vi "_script_execute.vi"(4 "QD Plugins Dir":path, 6 "QD Text":string, 8 "error in (no error)":errorcluster, 9 "Shift?":bool, 10 "Focus":enum8{"FP", "BD"}(ring), 11 "VI Refnum":refnum<vi>) -> (0 "error out":errorcluster)   [LabVIEW 2019, in "Script.lvlib"]
doc: "Executes scripts shortcuts defined in the Quick Drop arguments.\n\nHelp: Ctrl-Space + \"?\" + Ctrl-S\n\nCreated by: Ryan Pacini"
uses:
  Script.lvlib
  _script_defs.ctl
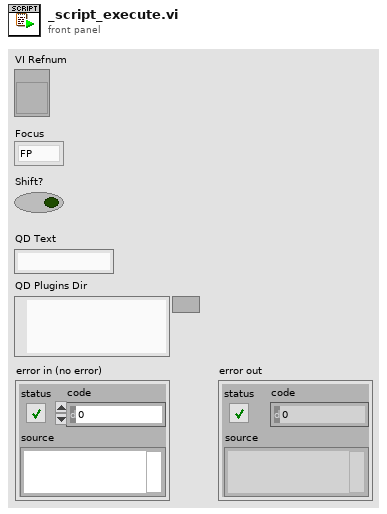
[diagram p1: front panel]
types:
  T1 = typedef "Script.lvlib/_script_defs.ctl" = cluster{"plugins":cluster{"vi":path, "desc":string}[], "defaults":cluster{"uid":string, "name":string}[], "shortcuts":cluster{"shortcut":string, "uids":string[]}[], "defaults?":bool}
  T2 = enum16{"open", "replace", "create", "open or create", "replace or create", "replace or create with confirmation"}
  T3 = cluster{"name":string, "default":cluster{"uid":string, "name":string}}
  T4 = cluster{"name":string, "default":cluster{"uid":string, "name":string}}[]
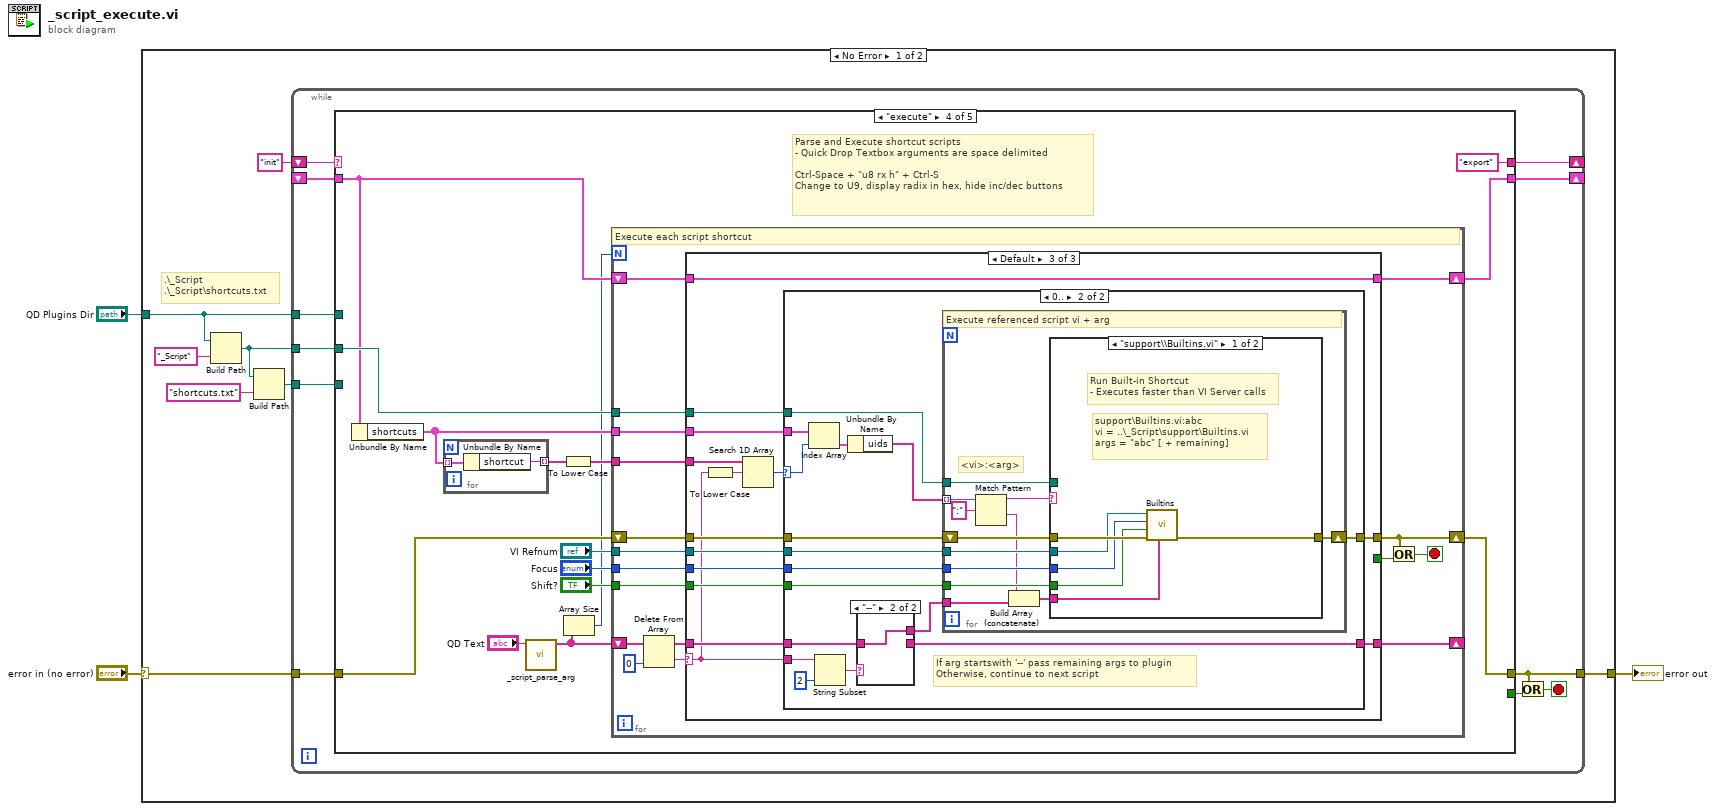
[diagram p0: block diagram]
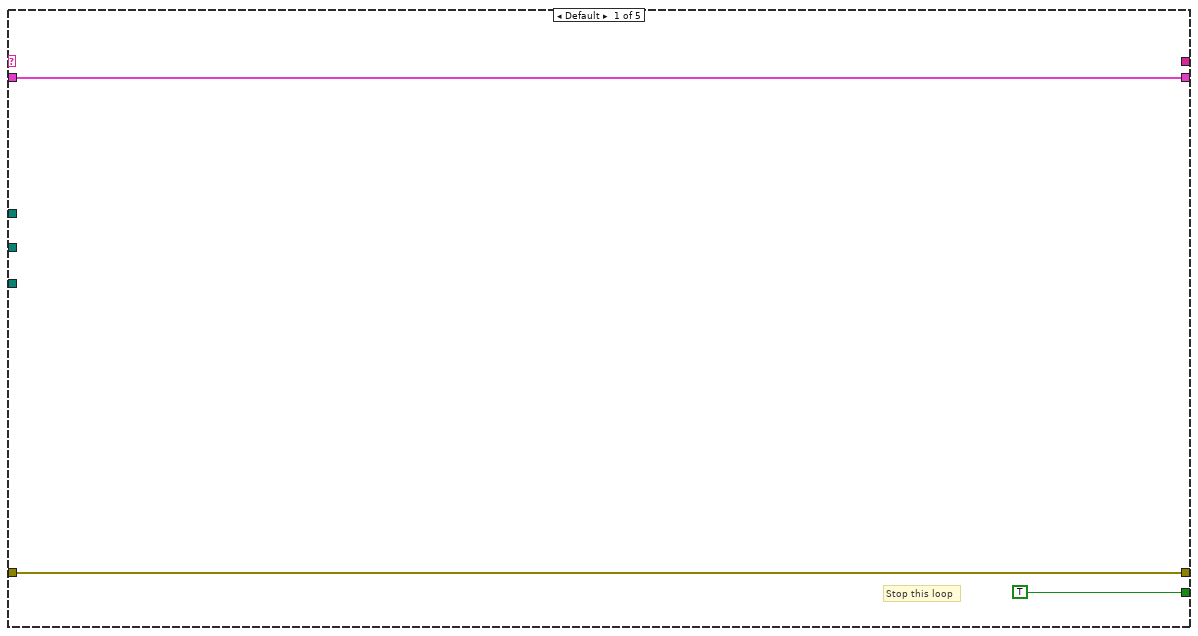
[diagram p2: hidden frame]
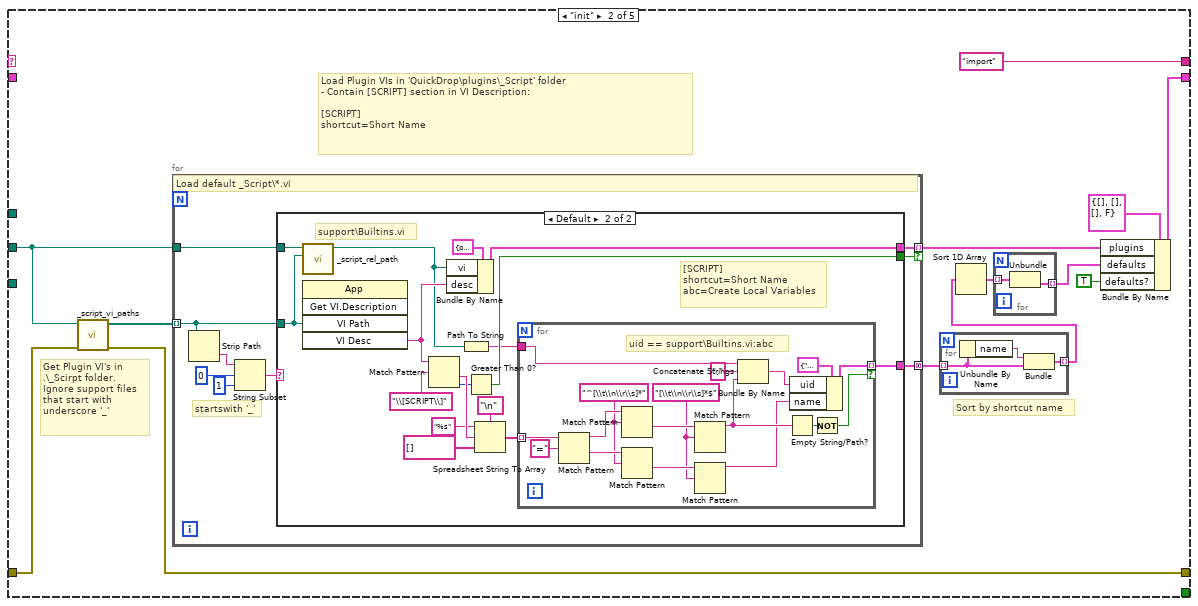
[diagram p3: hidden frame]
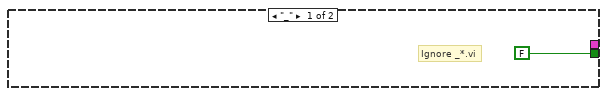
[diagram p4: hidden frame]
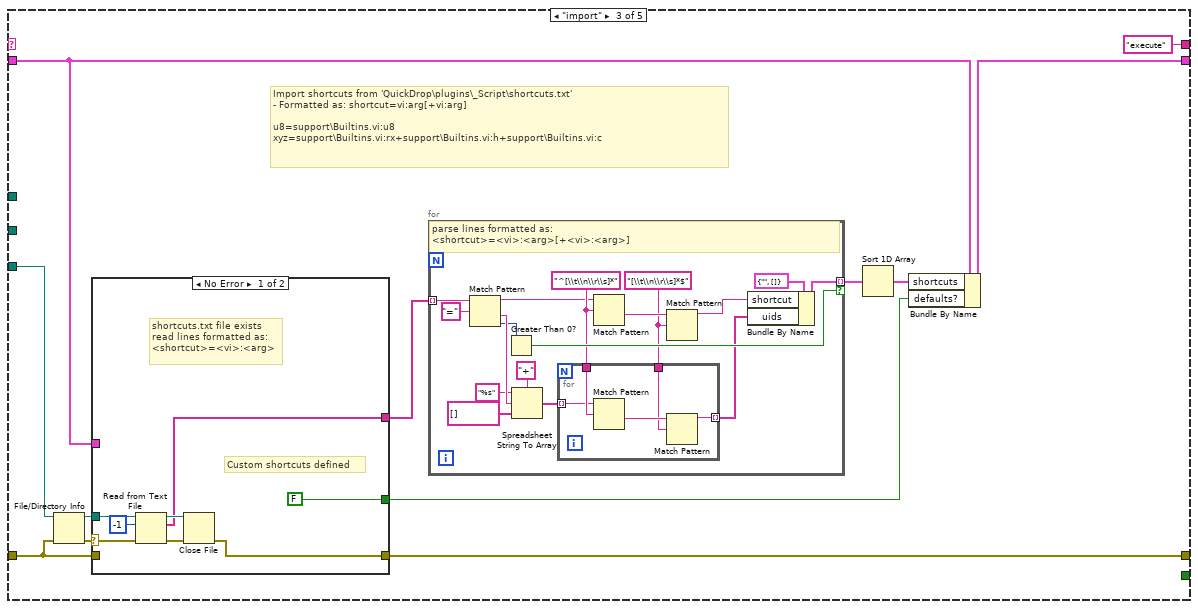
[diagram p5: hidden frame]
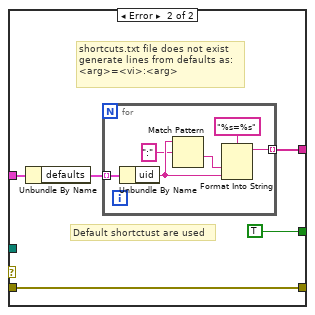
[diagram p6: hidden frame]
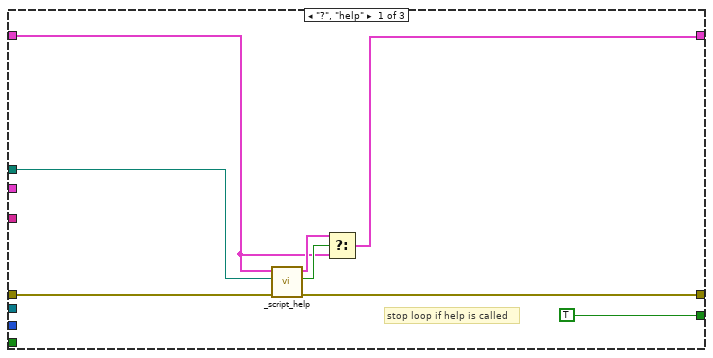
[diagram p7: hidden frame]
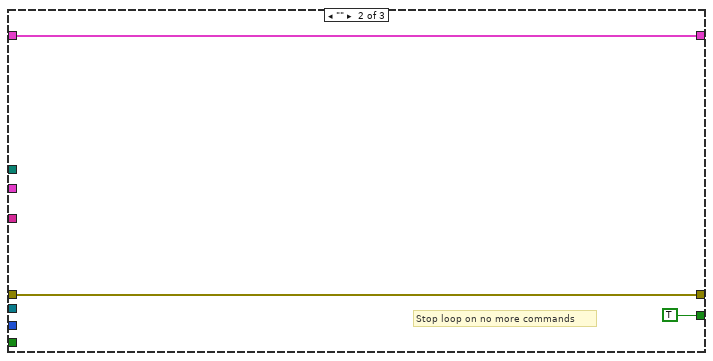
[diagram p8: hidden frame]
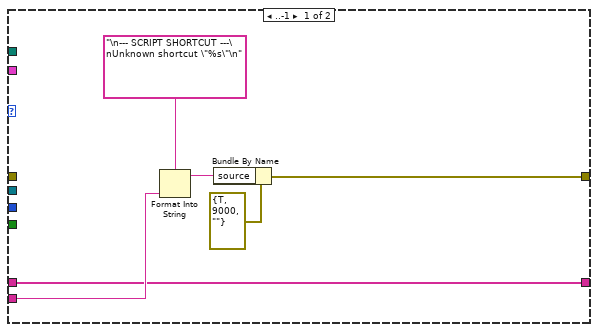
[diagram p9: hidden frame]
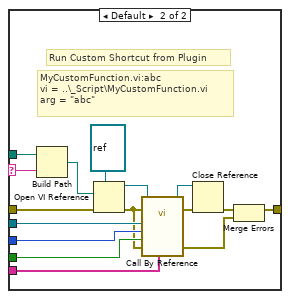
[diagram p11: hidden frame]
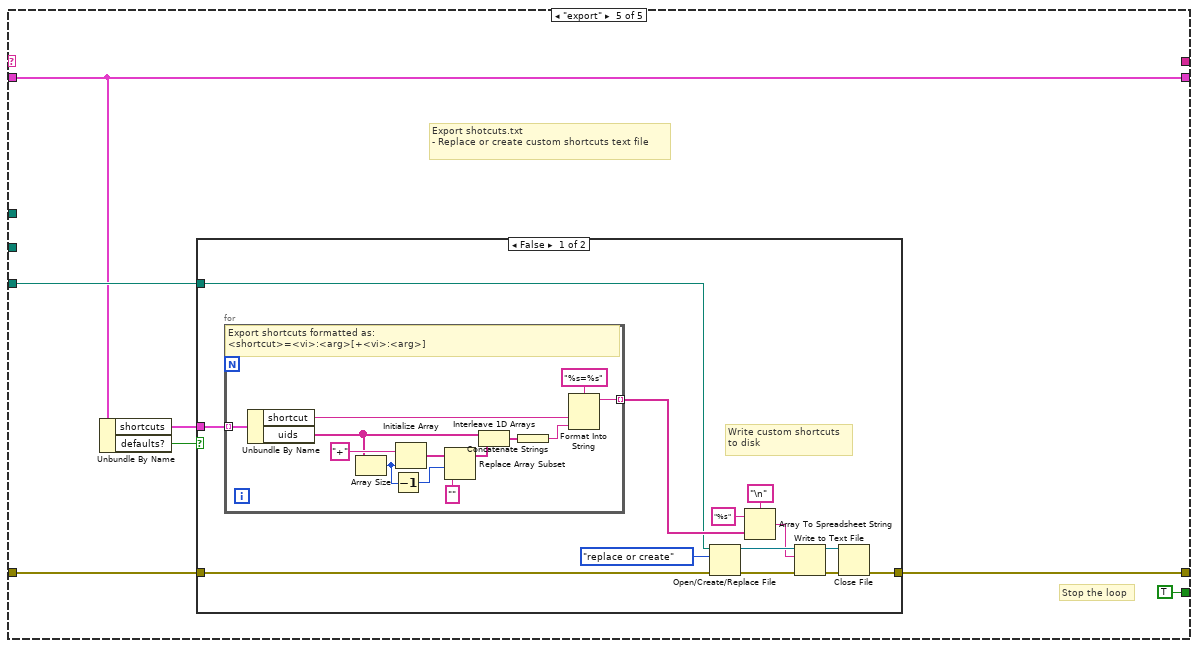
[diagram p12: hidden frame]
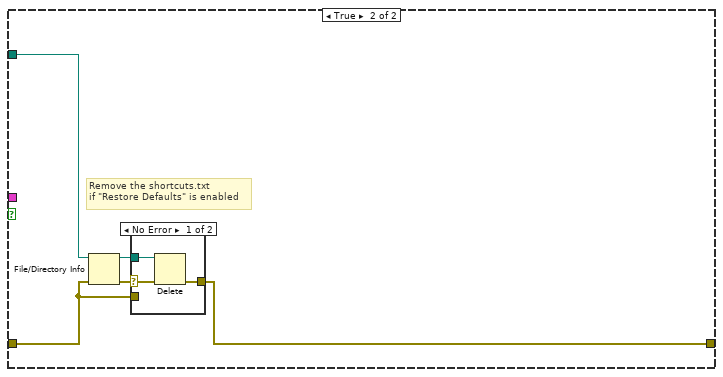
[diagram p13: hidden frame]
diagram:
  n1 = case shown="No Error" "error in (no error)" {
    selector: "error in (no error)" -> [w10 w299]
    tunnel: [w8 w299] -> w2
    tunnel: "QD Plugins Dir" -> [w6 _]
    frame No Error {
      # ".\\_Script\n.\\_Script\\shortcuts.txt"
      n2 = Build Path(base path=w6, name or relative path="_Script") -> (appended path=w5:path)
      n3 = Build Path(base path=w5, name or relative path="shortcuts.txt") -> (appended path=w4:path)
      n4 = while {
        tunnel: w10 -> [w22]
        tunnel: w5 -> [w21]
        shift-right: [w19] -> _
        shift-left: "init" -> [w20]
        shift-right: [w18] -> _
        shift-left: _ -> [w17]
        tunnel: [w16] -> w8
        tunnel: w6 -> [w13]
        tunnel: w4 -> [w12]
        stop <- w15 stop-if-true
        n5 = case shown="\"execute\"" w20 {
          tunnel: w22 -> [w24 w30 w94 w154 w263]
          tunnel: w21 -> [_ w27 _ w147 _]
          tunnel: [_ "import" "execute" "export" _] -> w19
          tunnel: [w25 w37 w91 w148 w260] -> w18
          tunnel: w17 -> [w25 _ w92 w143 w260]
          tunnel: [w24 w29 w98 w150 w262] -> w16
          tunnel: [TRUE _ _ _ TRUE] -> w14
          tunnel: w13 -> [_ _ _ _ _]
          tunnel: w12 -> [_ _ w93 _ w261]
          frame Default {
            # "Stop this loop"
          }
          frame "init" {
            # "Load Plugin VIs in 'QuickDrop\\plugins\\_Script' folder\n- Contain [SCRIPT] section in VI Description:\n\n[SCRIPT]\nshortcut=Short Name"
            # "Get Plugin VI's in \n.\\_Scirpt folder.\nIgnore support files \nthat start with\nunderscore '_'"
            # "Sort by shortcut name"
            n6 = call "_script_vi_paths.vi"("error in (no error)"=w30, "Directory"=w27) -> ("error out"=w29:errorcluster, "VI Paths"=w28:path[])  [unwired: 8 in]
            n7 = for {
              tunnel: w28 -> [w52] mode=indexing
              tunnel: [w48] -> w35 mode=indexing if=w46
              tunnel: w27 -> [w45]
              tunnel: [w44] -> w34 mode=concatenating
              # "startswith '_'"
              # "Load default _Script\\*.vi"
              n8 = Strip Path(path=w52) -> (name=w51:string)  [unwired: 1 out]
              n9 = String Subset(string=w51, offset (0)=0, length (rest)=1 ("length (rest)")) -> (substring=w47:string)
              n10 = case shown="Default" w47 {
                tunnel: w52 -> [_ w55]
                tunnel: [_ w60] -> w48
                tunnel: [FALSE w62] -> w46
                tunnel: w45 -> [_ w56]
                tunnel: [_ w57] -> w44
                frame "_" {
                  # "Ignore _*.vi"
                }
                frame Default {
                  # "support\\Builtins.vi"
                  # "[SCRIPT]\nshortcut=Short Name\nabc=Create Local Variables"
                  n11 = call "_script_rel_path.vi"("Child"=w55, "Parent"=w56) -> ("Child Relative Path"=w54:path)  [unwired: 9 in]
                  n12 = invoke class="App" method="Get VI.Description"("VI Path"=w55) -> ("VI Desc"=w59:string)  [unwired: 4 in, 4 out]
                  n13 = Match Pattern(string=w59, regular expression="\\[SCRIPT\\]") -> (after substring=w68:string, offset past match=w63:i32)  [unwired: 1 in, 2 out]
                  n14 = Bundle By Name(cluster=cluster{"vi":path, "desc":string} {"vi"=path "", "desc"=""} ("plugin"), "vi"=w54, "desc"=w59) -> (w60:cluster{"vi":path, "desc":string})
                  n15 = Path To String(path=w54) -> (string=w58:string)
                  n16 = Greater Than 0?(x=w63) -> (x > 0?=w62:bool)
                  n17 = Spreadsheet String To Array(delimiter (Tab)="\n", format string="%s", spreadsheet string=w68, array type (2D Dbl)=string[] []) -> (array=w64:string[])
                  n18 = for {
                    tunnel: w64 -> [w86] mode=indexing
                    tunnel: [w71] -> w57 mode=indexing if=w77
                    tunnel: w58 -> [w75]
                    w79 = "[\\t\\n\\r\\s]*$" ("regular expression")
                    w80 = "^[\\t\\n\\r\\s]*" ("regular expression")
                    # "uid == support\\Builtins.vi:abc"
                    n19 = Match Pattern(string=w86, regular expression="=") -> (before substring=w83:string, after substring=w81:string)  [unwired: 1 in, 2 out]
                    n20 = Match Pattern(string=w83, regular expression=w80) -> (after substring=w84:string)  [unwired: 1 in, 3 out]
                    n21 = Match Pattern(string=w81, regular expression=w80) -> (after substring=w82:string)  [unwired: 1 in, 3 out]
                    n22 = Match Pattern(string=w84, regular expression=w79) -> (before substring=w74:string)  [unwired: 1 in, 3 out]
                    n23 = Match Pattern(string=w82, regular expression=w79) -> (before substring=w70:string)  [unwired: 1 in, 3 out]
                    n24 = Concatenate Strings(w75, ":" ("string"), w74) -> (w72:string)
                    n25 = Empty String/Path?(string/path=w74) -> (empty?=w78:bool)
                    n26 = Bundle By Name(cluster=cluster{"uid":string, "name":string} {"uid"="", "name"=""} ("default"), "uid"=w72, "name"=w70) -> (w71:cluster{"uid":string, "name":string})
                    n27 = Not(x=w78) -> (.not. x?=w77:bool)
                  }
                }
              }
            }
            n28 = for {
              tunnel: w34 -> [w42] mode=indexing
              tunnel: [w41] -> w33 mode=indexing
              n29 = Unbundle By Name(w42) -> ("name"=w43:string)
              n30 = Bundle("name"=w43, "default"=w42) -> (w41:T3)  [unwired: 1 in]
            }
            n31 = Sort 1D Array(array=w33) -> (sorted array=w32:T4)
            n32 = for {
              tunnel: w32 -> [w40] mode=indexing
              tunnel: [w39] -> w31 mode=indexing
              n33 = Unbundle(w40) -> ("default"=w39:cluster{"uid":string, "name":string})  [unwired: 1 out]
            }
            n34 = Bundle By Name(cluster=T1 {"plugins"=[], "defaults"=[], "shortcuts"=[], "defaults?"=FALSE} ("data"), "plugins"=w35, "defaults"=w31, "defaults?"=TRUE) -> (w37:T1)
          }
          frame "import" {
            # "Import shortcuts from 'QuickDrop\\plugins\\_Script\\shortcuts.txt'\n- Formatted as: shortcut=vi:arg[+vi:arg]\n\nu8=support\\Builtins.vi:u8\nxyz=support\\Builtins.vi:rx+support\\Builtins.vi:h+support\\Builtins.vi:c"
            n35 = File/Directory Info(path=w93, error in=w94) -> (path out=w97:path, error out=w96:errorcluster)  [unwired: 5 out]
            n36 = case shown="No Error" w96 {
              selector: w96 -> [w105 _]
              tunnel: [w101 w108] -> w98
              tunnel: w97 -> [w106 _]
              tunnel: w92 -> [_ w110]
              tunnel: w94 -> [_ w108]
              tunnel: [w100 w109] -> w95
              tunnel: [FALSE TRUE] -> w87
              frame No Error {
                # "Custom shortcuts defined"
                # "shortcuts.txt file exists\nread lines formatted as:\n<shortcut>=<vi>:<arg>"
                n37 = Read from Text File(file (use dialog)=w106, count=-1, error in=w105) -> (refnum out=w102:refnum<file>, text=w100:string[], error out=w103:errorcluster)  [unwired: 1 in, 1 out]
                n38 = Close File(refnum=w102, error in=w103) -> (error out=w101:errorcluster)  [unwired: 1 out]
              }
              frame Error {
                # "Default shortctust are used"
                # "shortcuts.txt file does not exist\ngenerate lines from defaults as:\n<arg>=<vi>:<arg>"
                n39 = Unbundle By Name(w110) -> ("defaults"=w111:cluster{"uid":string, "name":string}[])
                n40 = for {
                  tunnel: w111 -> [w117] mode=indexing
                  tunnel: [w116] -> w109 mode=indexing
                  n41 = Unbundle By Name(w117) -> ("uid"=w114:string)
                  n42 = Match Pattern(string=w114, regular expression=":") -> (after substring=w112:string)  [unwired: 1 in, 3 out]
                  n43 = Format Into String(format string="%s=%s", w112, w114) -> (resulting string=w116:string)  [unwired: 2 in, 1 out]
                }
              }
            }
            n44 = for {
              tunnel: w95 -> [w134] mode=indexing
              tunnel: [w125] -> w89 mode=indexing if=w127
              w122 = "[\\t\\n\\r\\s]*$" ("regular expression")
              w123 = "^[\\t\\n\\r\\s]*" ("regular expression")
              # "parse lines formatted as:\n<shortcut>=<vi>:<arg>[+<vi>:<arg>]"
              n45 = Match Pattern(string=w134, regular expression="=") -> (before substring=w121:string, after substring=w132:string, offset past match=w128:i32)  [unwired: 1 in, 1 out]
              n46 = Greater Than 0?(x=w128) -> (x > 0?=w127:bool)
              n47 = Spreadsheet String To Array(delimiter (Tab)="+", format string="%s", spreadsheet string=w132, array type (2D Dbl)=string[] []) -> (array=w119:string[])
              n48 = for {
                tunnel: w123 -> [w138]
                tunnel: w122 -> [w137]
                tunnel: w119 -> [w136] mode=indexing
                tunnel: [w135] -> w118 mode=indexing
                n49 = Match Pattern(string=w136, regular expression=w138) -> (after substring=w139:string)  [unwired: 1 in, 3 out]
                n50 = Match Pattern(string=w139, regular expression=w137) -> (before substring=w135:string)  [unwired: 1 in, 3 out]
              }
              n51 = Match Pattern(string=w121, regular expression=w123) -> (after substring=w124:string)  [unwired: 1 in, 3 out]
              n52 = Match Pattern(string=w124, regular expression=w122) -> (before substring=w120:string)  [unwired: 1 in, 3 out]
              n53 = Bundle By Name(cluster=cluster{"shortcut":string, "uids":string[]} {"shortcut"="", "uids"=[]} ("shortcut"), "shortcut"=w120, "uids"=w118) -> (w125:cluster{"shortcut":string, "uids":string[]})
            }
            n54 = Sort 1D Array(array=w89) -> (sorted array=w88:cluster{"shortcut":string, "uids":string[]}[])
            n55 = Bundle By Name(cluster=w92, "shortcuts"=w88, "defaults?"=w87) -> (w91:T1)
          }
          frame "execute" {
            # "Parse and Execute shortcut scripts\n- Quick Drop Textbox arguments are space delimited\n\nCtrl-Space + \"u8 rx h\" + Ctrl-S\nChange to U9, display radix in hex, hide inc/dec buttons"
            n56 = Unbundle By Name(w143) -> ("shortcuts"=w144:cluster{"shortcut":string, "uids":string[]}[])
            n57 = for {
              tunnel: w144 -> [w256] mode=indexing
              tunnel: [w255] -> w146 mode=indexing
              n58 = Unbundle By Name(w256) -> ("shortcut"=w255:string)
            }
            n59 = call "_script_parse_arg.vi"("QD Text"="QD Text") -> ("args"=w140:string[])  [unwired: 10 in]
            n60 = To Lower Case(string=w146) -> (all lower case string=w145:string[])
            n61 = Array Size(array=w140) -> (size(s)=w141:i32)
            n62 = for {
              N: w141 -> [_]
              tunnel: w145 -> [w171]
              tunnel: w144 -> [w170]
              tunnel: "VI Refnum" -> [w168]
              tunnel: "Focus" -> [w167]
              tunnel: "Shift?" -> [w166]
              shift-right: [w162] -> w150
              shift-left: w154 -> [w169]
              shift-right: [w165] -> w148
              shift-left: w143 -> [w164]
              tunnel: w147 -> [w163]
              shift-right: [w156] -> _
              shift-left: w140 -> [w160]
              stop <- w158 stop-if-true
              # "Execute each script shortcut"
              n63 = Delete From Array(array=w160, index=0) -> (deleted portion=w155:string, array with subset deleted=w157:string[])  [unwired: 1 in]
              n64 = case shown="Default" w155 {
                selector: w155 -> [_ _ w184]
                tunnel: w171 -> [_ _ w196]
                tunnel: w170 -> [_ _ w194]
                tunnel: w169 -> [w179 w181 w193]
                tunnel: w168 -> [_ _ w192]
                tunnel: w167 -> [_ _ w191]
                tunnel: w166 -> [_ _ w190]
                tunnel: [w178 w181 w189] -> w162
                tunnel: [w174 w182 w188] -> w165
                tunnel: w164 -> [w175 w182 w188]
                tunnel: w163 -> [w173 _ w187]
                tunnel: [TRUE TRUE _] -> w161
                tunnel: w157 -> [_ _ w186]
                tunnel: [_ _ w185] -> w156
                frame "?", "help" {
                  # "stop loop if help is called"
                  n65 = call "_script_help.vi"("error in (no error)"=w179, "_Script Dir"=w173, "Definitions in"=w175) -> ("error out"=w178:errorcluster, "commit?"=w177:bool, "Definitions out"=w176:T1)  [unwired: 6 in]
                  n66 = Select(t=w176, s=w177, f=w175) -> (s? t:f=w174:T1)
                }
                frame "" {
                  # "Stop loop on no more commands"
                }
                frame Default {
                  n67 = To Lower Case(string=w184) -> (all lower case string=w183:string)
                  n68 = Search 1D Array(1D array=w196, element=w183) -> (index of element=w195:i32)  [unwired: 1 in]
                  n69 = case shown="0.." w195 {
                    selector: w195 -> [_ w218]
                    tunnel: w194 -> [_ w217]
                    tunnel: w193 -> [_ w214]
                    tunnel: w192 -> [_ w213]
                    tunnel: w191 -> [_ w212]
                    tunnel: w190 -> [_ w211]
                    tunnel: [w201 w210] -> w189
                    tunnel: w187 -> [_ w209]
                    tunnel: w184 -> [w200 w207]
                    tunnel: w186 -> [w197 w205]
                    tunnel: [w197 w204] -> w185
                    frame ..-1 {
                      n70 = Format Into String(format string="\n--- SCRIPT SHORTCUT ---\nUnknown shortcut \"%s\"\n" ("source"), w200) -> (resulting string=w198:string)  [unwired: 2 in, 1 out]
                      n71 = Bundle By Name(cluster=errorcluster {"status"=TRUE, "code"=9000, "source"=""} ("error IO"), "source"=w198) -> (w201:errorcluster)
                    }
                    frame 0.. {
                      # "If arg startswith '--' pass remaining args to plugin\nOtherwise, continue to next script"
                      n72 = Index Array(array=w217, index=w218) -> (element=w216:cluster{"shortcut":string, "uids":string[]})
                      n73 = String Subset(string=w207, length (rest)=2 ("length (rest)")) -> (substring=w206:string)  [unwired: 1 in]
                      n74 = Unbundle By Name(w216) -> ("uids"=w215:string[])
                      n75 = case shown="\"--\"" w206 {
                        tunnel: w205 -> [w219 w220]
                        tunnel: [w219 _] -> w204
                        tunnel: [_ w220] -> w203
                        frame Default {
                        }
                        frame "--" {
                        }
                      }
                      n76 = for {
                        tunnel: w215 -> [w226] mode=indexing
                        tunnel: w213 -> [w231]
                        tunnel: w212 -> [w230]
                        tunnel: w211 -> [w229]
                        shift-right: [w228] -> w210
                        shift-left: w214 -> [w232]
                        tunnel: w209 -> [w223]
                        tunnel: w203 -> [w222]
                        # "<vi>:<arg>"
                        # "Execute referenced script vi + arg"
                        n77 = Match Pattern(string=w226, regular expression=":") -> (before substring=w224:string, after substring=w227:string)  [unwired: 1 in, 2 out]
                        n78 = Build Array (concatenate)(w227, w222) -> (w221:string[])
                        n79 = case shown="\"support\\\\Builtins.vi\"" w224 {
                          selector: w224 -> [_ w242]
                          tunnel: w232 -> [w238 w254]
                          tunnel: w231 -> [w237 w251]
                          tunnel: w230 -> [w236 w250]
                          tunnel: w229 -> [w235 w249]
                          tunnel: [w234 w244] -> w228
                          tunnel: w223 -> [_ w241]
                          tunnel: w221 -> [w233 w239]
                          frame "support\\Builtins.vi" {
                            # "support\\Builtins.vi:abc\nvi = ..\\_Script\\support\\Builtins.vi\nargs = \"abc\" [ + remaining]"
                            # "Run Built-in Shortcut\n- Executes faster than VI Server calls"
                            n80 = call "Builtins.vi"("args"=w233, "error in (no error)"=w238, "Shift?"=w235, "Focus"=w236, "VI Refnum"=w237) -> ("error out"=w234:errorcluster)  [unwired: 6 in]
                          }
                          frame Default {
                            # "Run Custom Shortcut from Plugin"
                            # "MyCustomFunction.vi:abc\nvi = ..\\_Script\\MyCustomFunction.vi\narg = \"abc\""
                            n81 = Build Path(base path=w241, name or relative path=w242) -> (appended path=w240:path)
                            n82 = Open VI Reference(type specifier VI Refnum (for type only)=refnum<vi> refnum, vi path=w240, error in (no error)=w254) -> (vi reference=w252:refnum<vi>, error out=w248:errorcluster)  [unwired: 3 in]
                            n83 = call-by-ref "?"(reference=w252, error in=w248, "args"=w239, 8:"error in (no error)"=w248, "Shift?"=w249, "Focus"=w250, "VI Refnum"=w251) -> (reference out=w246:refnum<vi>, error out=w247:errorcluster, 0:"error out"=w243:errorcluster)  [unwired: 6 in]
                            n84 = Close Reference(reference=w246, error in (no error)=w247) -> (error out=w245:errorcluster)
                            n85 = Merge Errors(w245, w243) -> (w244:errorcluster)
                          }
                        }
                      }
                    }
                  }
                }
              }
              n86 = Or(x=w162, y=w161) -> (x .or. y?=w158:bool)
            }
          }
          frame "export" {
            # "Export shotcuts.txt\n- Replace or create custom shortcuts text file"
            # "Stop the loop"
            n87 = Unbundle By Name(w260) -> ("shortcuts"=w259:cluster{"shortcut":string, "uids":string[]}[], "defaults?"=w257:bool)
            n88 = case shown="False" w257 {
              tunnel: w263 -> [w276 w290]
              tunnel: [w266 w291] -> w262
              tunnel: w261 -> [w265 w294]
              tunnel: w259 -> [w264 _]
              frame False {
                # "Write custom shortcuts\nto disk"
                n89 = for {
                  tunnel: [w289] -> w275 mode=indexing
                  tunnel: w264 -> [w288] mode=indexing
                  # "Export shortcuts formatted as:\n<shortcut>=<vi>:<arg>[+<vi>:<arg>]"
                  n90 = Unbundle By Name(w288) -> ("shortcut"=w287:string, "uids"=w278:string[])
                  n91 = Array Size(array=w278) -> (size(s)=w283:i32)
                  n92 = Decrement(x=w283) -> (x-1=w282:i32)
                  n93 = Initialize Array("+" ("delimiter (Tab)"), w283) -> (w284:string[])
                  n94 = Replace Array Subset(array=w284, new element="" ("new element/subarray"), index=w282) -> (w281:string[])
                  n95 = Interleave 1D Arrays(w278, w281) -> (w279:string[])
                  n96 = Concatenate Strings(w279) -> (w277:string)
                  n97 = Format Into String(format string="%s=%s", w287, w277) -> (resulting string=w289:string)  [unwired: 2 in, 1 out]
                }
                n98 = Open/Create/Replace File(file path (use dialog)=w265, error in=w276, operation (0:open)=T2."replace or create") -> (refnum out=w273:refnum<file>, error out=w274:errorcluster)  [unwired: 3 in, 1 out]
                n99 = Array To Spreadsheet String(delimiter (Tab)="\n", array=w275, 3:"%s" ("format string")) -> (spreadsheet string=w267:string)
                n100 = Write to Text File(file (use dialog)=w273, text=w267, error in=w274) -> (refnum out=w272:refnum<file>, error out=w271:errorcluster)  [unwired: 1 in, 1 out]
                n101 = Close File(refnum=w272, error in=w271) -> (error out=w266:errorcluster)  [unwired: 1 out]
              }
              frame True {
                # "Remove the shortcuts.txt\nif \"Restore Defaults\" is enabled"
                n102 = File/Directory Info(path=w294, error in=w290) -> (path out=w292:path, error out=w293:errorcluster)  [unwired: 5 out]
                n103 = case shown="No Error" w293 {
                  selector: w293 -> [w297 _]
                  tunnel: w292 -> [w296 _]
                  tunnel: [w295 w298] -> w291
                  tunnel: w290 -> [_ w298]
                  frame No Error {
                    n104 = Delete(path (use dialog)=w296, error in=w297) -> (error out=w295:errorcluster)  [unwired: 3 in, 2 out]
                  }
                  frame Error {
                  }
                }
              }
            }
          }
        }
        n105 = Or(x=w16, y=w14) -> (x .or. y?=w15:bool)
      }
    }
    frame Error {
    }
  }
  "error out" <- w2
